vi "IsValid.vi"(8 "error in (no error)":errorcluster, 11 "Link in":refnum<class "Link.lvclass">) -> (0 "error out":errorcluster, 2 "valid":bool, 3 "Link out":refnum<class "Link.lvclass">)   [LabVIEW 2009, in "NavScreen.lvlib" / "Link.lvclass"]
uses:
  Link.lvclass
  Link.lvclass/Link.ctl
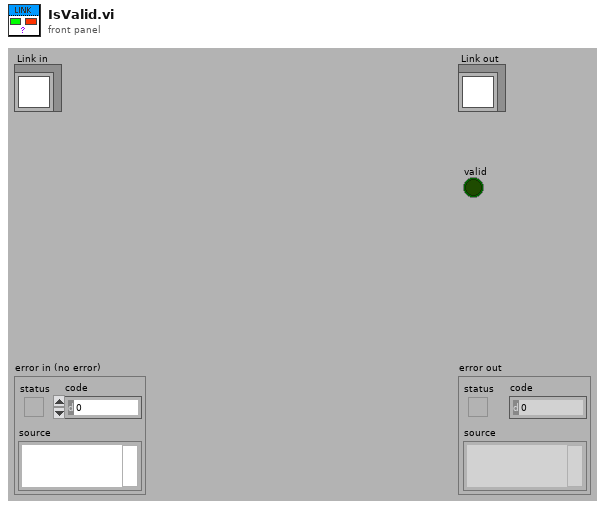
[diagram p1: front panel]
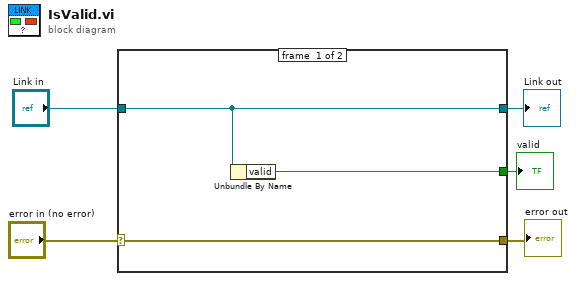
[diagram p0: block diagram]
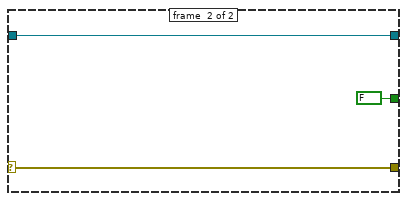
[diagram p2: hidden frame]
diagram:
  n1 = case shown="No Error" "error in (no error)" {
    selector: "error in (no error)" -> [w8 w11]
    tunnel: [w8 w11] -> w4
    tunnel: [w7 w10] -> w2
    tunnel: "Link in" -> [w7 w10]
    tunnel: [w6 FALSE ("valid")] -> w1
    frame #0 {
      n2 = Unbundle By Name(w7) -> ("valid"=w6:bool)
    }
    frame #1 {
    }
  }
  "error out" <- w4
  "Link out" <- w2
  "valid" <- w1
